vi "Fixed-Point Configuration.vi"() -> ()   [LabVIEW 2012]
uses:
  <vilib>/rvi/eio/common/nirviEmuTemplateMethod_errors.vi
  <vilib>/eio/EIONode/EIONode.xnode
panel:
  out "Simulated AI0":fxp<+/-,24,4>
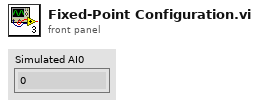
[diagram p1: front panel]
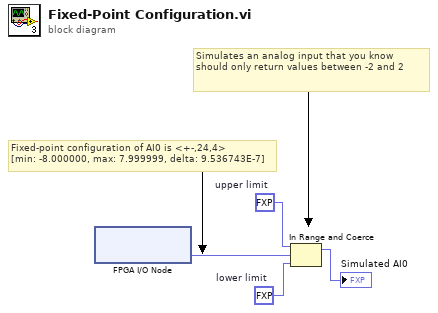
[diagram p0: block diagram]
diagram:
  w2 = fxp<+/-,24,4> -2.0  # lower limit
  w3 = fxp<+/-,24,4> 2.0  # upper limit
  # "Simulates an analog input that you know should only return values between -2 and 2"
  # "Fixed-point configuration of AI0 is <+-,24,4>\n[min: -8.000000, max: 7.999999, delta: 9.536743E-7]"
  n1 = xnode "FPGA I/O Node"() -> ("Mod2/AI0"=w4:fxp<+/-,24,4>)  [unwired: 1 in, 1 out]
  n2 = In Range and Coerce(upper limit=w3, x=w4, lower limit=w2) -> (coerced(x)=→"Simulated AI0":fxp<+/-,24,4>)  [unwired: 1 out]
